vi "PV ActiveLine - Gas Type Correction.vi"   [LabVIEW 2013, in "PV ActiveLine.lvlib"]
uses:
  <instrlib>/PV ActiveLine/PV ActiveLine.lvlib
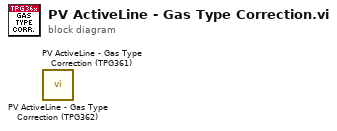
[diagram p0: block diagram]
diagram:
  n1 = call <instrlib>:"PV ActiveLine - Gas Type Correction (TPG362).vi"() -> ()  [unwired: 8 in, 4 out]
  n2 = call <instrlib>:"PV ActiveLine - Gas Type Correction (TPG361).vi"() -> ()  [unwired: 9 in, 3 out]
